vi "Enable_Disable Stream.vi"(7 "time":i16=10, 8 "error in":errorcluster, 9 "Enable?":bool, 10 "String":string="ZDA", 11 "Airmar WS in":refnum<class "Airmar WS.lvclass">) -> (0 "error out":errorcluster, 3 "Airmar WS out":refnum<class "Airmar WS.lvclass">)   [LabVIEW 2014, in "Airmar WS.lvclass"]
uses:
  Airmar WS.lvclass
  Airmar WS.lvclass/Airmar WS.ctl
  Reusable/Session APIs/Text Communication/Text Device Session.lvclass
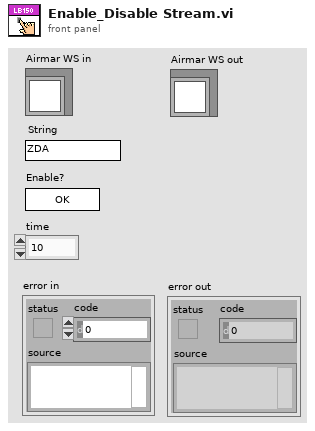
[diagram p1: front panel]
types:
  T1 = typedef "Session - Root.lvclass/Session Handle.ctl" = refnum<data-value>
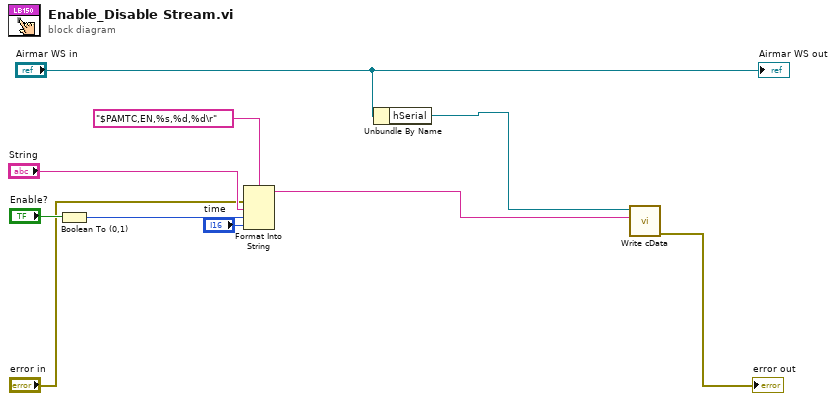
[diagram p0: block diagram]
diagram:
  n1 = Boolean To (0,1)(Boolean="Enable?") -> (0, 1=w7:i16)
  n2 = Format Into String(format string="$PAMTC,EN,%s,%d,%d\r", error in="error in", "String", w7, "time") -> (resulting string=w2:string)  [unwired: 1 in, 1 out]
  n3 = Unbundle By Name("Airmar WS in") -> ("hSerial"=w3:T1)
  n4 = call "Write cData.vi"("Data"=w2, "hSession In"=w3) -> ("error out"=→"error out":errorcluster)  [unwired: 8 in, 1 out]
  "Airmar WS out" <- "Airmar WS in"
